vi "TcA01-001_ObjectCreationAndDestructionOfBaseclass.vi"(1 "Input buffer":T3="1", 3 "Invocation info":T2, 5 "error in (no error)":errorcluster, 6 "Add log to result?":bool) -> (16 "Test Data":T1 {"Numeric Measurement" format="%.2f"}, 19 "error out":errorcluster)   [LabVIEW 2009]
doc: "Test case template."
uses:
  Shared/Support_InputBuffer.ctl
  Shared/Support_InvocationInfo.ctl
  Shared/Support_TestData.ctl
  TestClasses/G#BaseClass1_class/G#BaseClass1.lvclass
  <vilib>/addons/_AddQ/G#Object/G#Object.lvclass
panel:
  in  "Test name":string="TcA01-001 Object creation and destruction of base class"
  out "Test result":bool
  out "Result":string
  # "Verify that multiple objects of a base class can\nbe created and destructed multiple times."
  # "Sub test case"
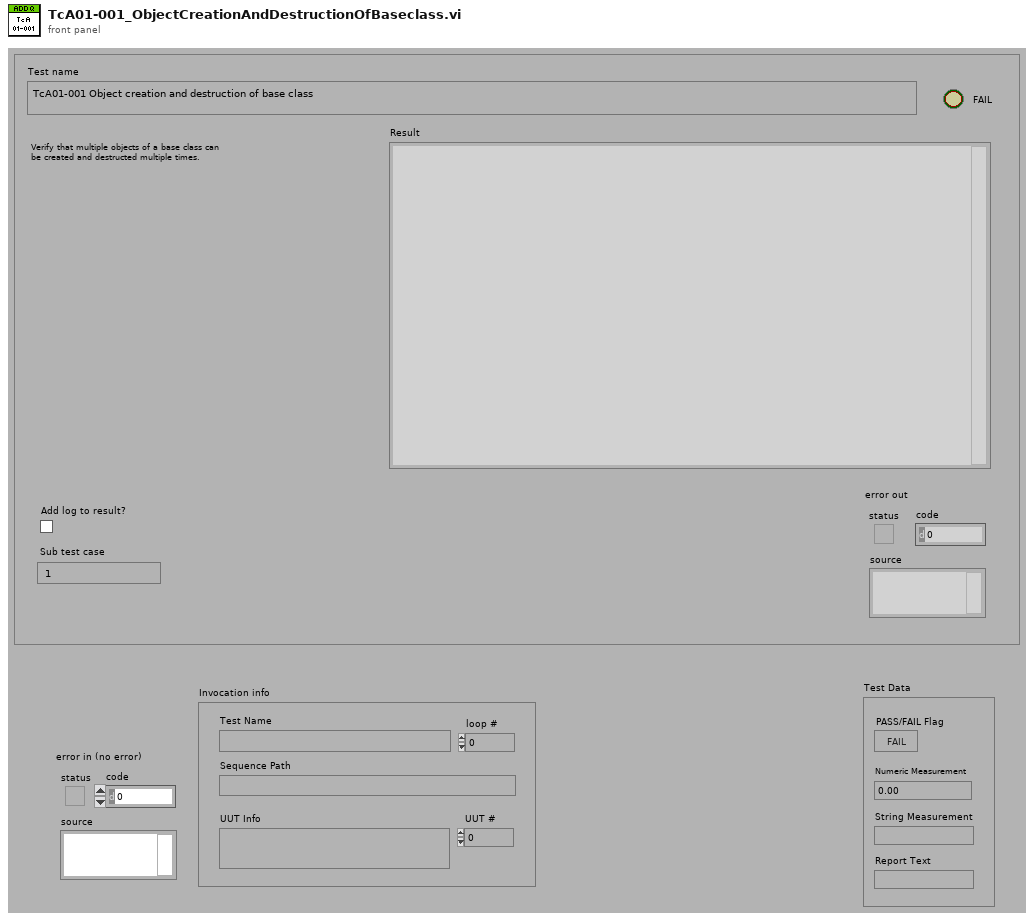
[diagram p1: front panel]
types:
  T1 = typedef "Support_TestData.ctl" = cluster{"PASS/FAIL Flag":bool, "Numeric Measurement":dbl, "String Measurement":string, "Report Text":string}
  T2 = typedef "Support_InvocationInfo.ctl" = cluster{"UUT #":i32, "loop #":i32, "UUT Info":string, "Test Name":string, "Sequence Path":path}
  T3 = typedef "Support_InputBuffer.ctl" = string
  T4 = typedef "Support_ResultType.ctl" = cluster{"Pass":bool, "Comment":string, "MeasurementValue":dbl}
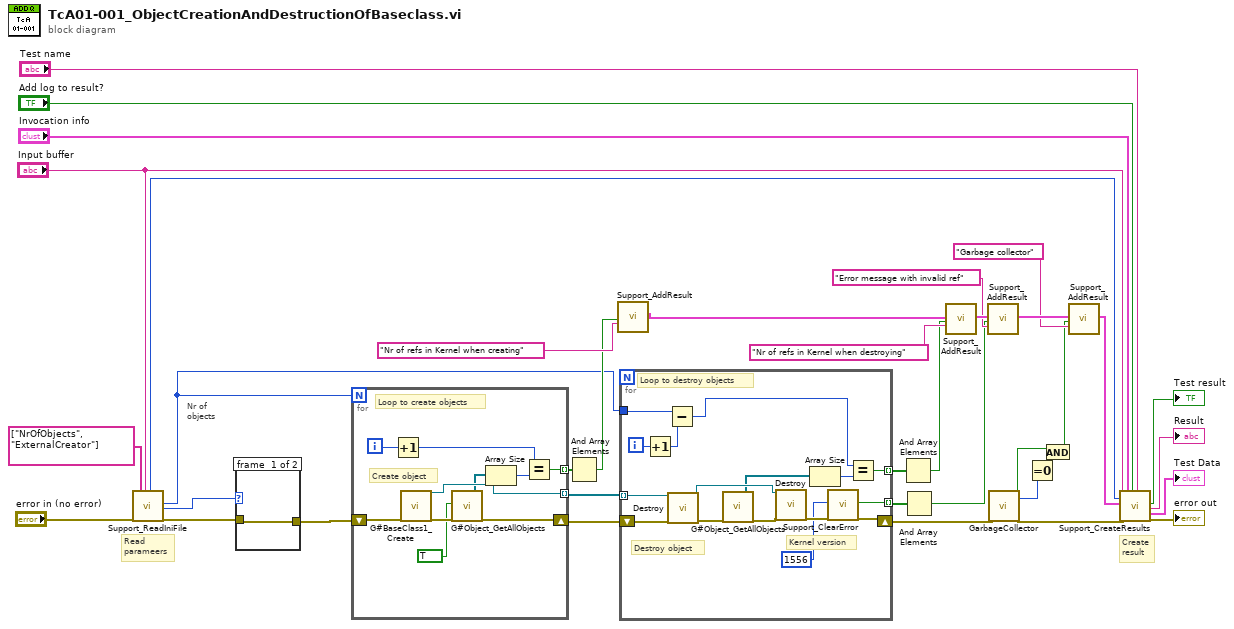
[diagram p0: block diagram]
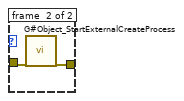
[diagram p2: hidden frame]
diagram:
  # "Read\nparameers"
  # "Create\nresult"
  # "Nr of\nobjects"
  n1 = call "Support_ReadIniFile.vi"("error in (no error)"="error in (no error)", "Parameter names"=string[] ["NrOfObjects", "ExternalCreator"], "Sub test case"="Input buffer") -> ("Timer start"=w19:u32, "Parameter1 as I32"=w25:i32, "Parameter2 as I32"=w1:i32, "error out"=w3:errorcluster)  [unwired: 9 in, 4 out]
  n2 = case shown="1" w1 {
    tunnel: w3 -> [w38 w40]
    tunnel: [w38 w39] -> w2
    frame #0 {
    }
    frame #1 {
      n3 = call <vilib>:"G#Object_StartExternalCreateProcess.vi"("error in (no error)"=w40) -> ("error out"=w39:errorcluster)  [unwired: 18 in]
    }
  }
  n4 = for {
    N: w25 -> [_]
    shift-right: [w41] -> w27
    shift-left: w2 -> [w50]
    tunnel: [w44] -> w26 mode=indexing
    tunnel: [w46] -> w30 mode=indexing
    i -> [w49]
    # "Create object"
    # "Loop to create objects"
    n5 = Increment(x=w49) -> (x+1=w47:i32)
    n6 = call "G#BaseClass1_Create.vi"("error in (no error)"=w50) -> ("reference out"=w44:refnum<class "G#BaseClass1.lvclass">, "error out"=w45:errorcluster)  [unwired: 16 in, 1 out]
    n7 = call <vilib>:"G#Object_GetAllObjects.vi"("only refs (F)"=TRUE ("only refs"), "error in (no error)"=w45) -> ("all refs"=w43:refnum<class "G#Object.lvclass">[], "error out"=w41:errorcluster)  [unwired: 14 in, 2 out]
    n8 = Array Size(array=w43) -> (size(s)=w48:i32)
    n9 = Equal?(x=w47, y=w48) -> (x = y?=w46:bool)
  }
  n10 = And Array Elements(Boolean array=w30) -> (logical AND=w28:bool)
  n11 = call "Support_AddResult.vi"("Pass"=w28, "Comment"="Nr of refs in Kernel when creating") -> ("Results out"=w14:T4[])  [unwired: 17 in]
  n12 = for {
    shift-right: [w56] -> w13
    shift-left: w27 -> [w64]
    tunnel: [w65] -> w24 mode=indexing
    tunnel: w26 -> [w60] mode=indexing
    tunnel: w25 -> [w63]
    tunnel: [w55] -> w18 mode=indexing
    i -> [w66]
    # "Destroy object"
    # "Loop to destroy objects"
    # "Kernel version"
    n13 = Increment(x=w66) -> (x+1=w62:i32)
    n14 = Subtract(x=w63, y=w62) -> (x-y=w61:i32)
    n15 = call-dynamic "Destroy.vi"("reference in"=w60, "error in (no error)"=w64) -> ("reference out"=w54:refnum<class "G#BaseClass1.lvclass">, "error out"=w51:errorcluster)  [unwired: 16 in]
    n16 = call <vilib>:"G#Object_GetAllObjects.vi"("error in (no error)"=w51) -> ("all refs"=w52:refnum<class "G#Object.lvclass">[], "error out"=w53:errorcluster)  [unwired: 15 in, 2 out]
    n17 = call-dynamic "Destroy.vi"("reference in"=w54, "error in (no error)"=w53) -> ("error out"=w58:errorcluster)  [unwired: 16 in, 1 out]
    n18 = Array Size(array=w52) -> (size(s)=w59:i32)
    n19 = call "Support_ClearError.vi"("code"=1556, "error in (no error)"=w58) -> ("Cleared?"=w55:bool, "error out"=w56:errorcluster)  [unwired: 16 in]
    n20 = Equal?(x=w61, y=w59) -> (x = y?=w65:bool)
  }
  n21 = And Array Elements(Boolean array=w24) -> (logical AND=w22:bool)
  n22 = And Array Elements(Boolean array=w18) -> (logical AND=w15:bool)
  n23 = call "Support_AddResult.vi"("Results in"=w14, "Pass"=w22, "Comment"="Nr of refs in Kernel when destroying") -> ("Results out"=w17:T4[])  [unwired: 16 in]
  n24 = call "Support_AddResult.vi"("Results in"=w17, "Pass"=w15, "Comment"="Error message with invalid ref") -> ("Results out"=w11:T4[])  [unwired: 16 in]
  n25 = call <vilib>:"GarbageCollector.vi"("error in (no error)"=w13) -> ("OK"=w8:bool, "# of objects killed"=w6:i32, "error out"=w12:errorcluster)  [unwired: 16 in]
  n26 = Equal To 0?(x=w6) -> (x = 0?=w7:bool)
  n27 = And(x=w8, y=w7) -> (x .and. y?=w5:bool)
  n28 = call "Support_AddResult.vi"("Results in"=w11, "Pass"=w5, "Comment"="Garbage collector") -> ("Results out"=w10:T4[])  [unwired: 16 in]
  n29 = call "Support_CreateResults.vi"("Sub test case"="Input buffer", "Timer start"=w19, "Results"=w10, "error in (no error)"=w12, "Invocation info"="Invocation info", "Add log to result?"="Add log to result?", "Test name"="Test name") -> ("Pass/fail flag"=→"Test result":bool, "Result"=→"Result":string, "Test Data"=→"Test Data":T1, "error out"=→"error out":errorcluster)  [unwired: 9 in]
